vi "Send.vi"(8 "error in (no error)":errorcluster, 10 "Message":string, 11 "Tovey9150 in":refnum<class "Tovey 9150.lvclass">) -> (0 "error out":errorcluster, 3 "Tovey9150 out":refnum<class "Tovey 9150.lvclass">)   [LabVIEW 2015, in "Tovey 9150.lvclass"]
uses:
  Tovey 9150.lvclass
  Tovey 9150.lvclass/Tovey 9150.ctl
  <userlib>/Common/SerialProtocols/SerialCommunicator/SerialCommunicator.lvclass
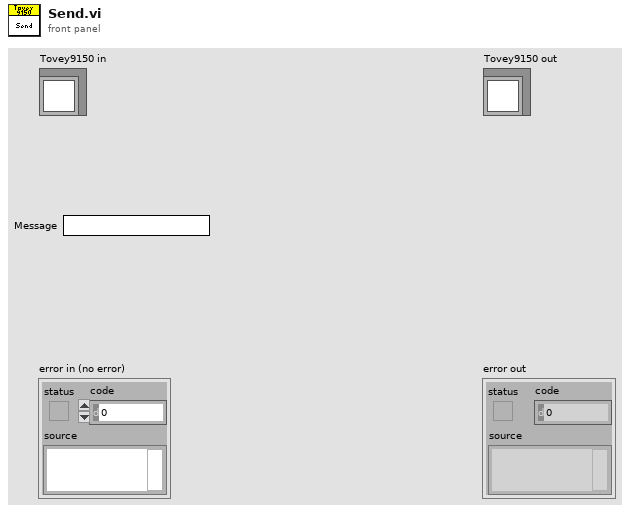
[diagram p1: front panel]
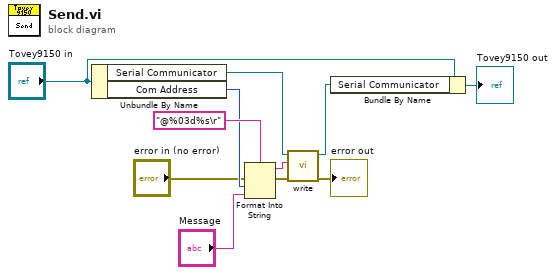
[diagram p0: block diagram]
diagram:
  n1 = Unbundle By Name("Tovey9150 in") -> ("Serial Communicator"=w11:refnum<class "SerialCommunicator.lvclass">, "Com Address"=w4:u8)
  n2 = Format Into String(format string="@%03d%s\r", error in="error in (no error)", w4, "Message") -> (resulting string=w3:string, error out=w1:errorcluster)  [unwired: 1 in]
  n3 = call-dynamic "write.vi"("error in (no error)"=w1, "writeString"=w3, "SerialCommunicator in"=w11) -> ("error out"=→"error out":errorcluster, "SerialCommunicator out"=w10:refnum<class "SerialCommunicator.lvclass">)  [unwired: 7 in]
  n4 = Bundle By Name(cluster="Tovey9150 in", "Serial Communicator"=w10) -> (→"Tovey9150 out":refnum<class "Tovey 9150.lvclass">)
